vi "ZK非断电保存全局变量.vi"() -> ()   [LabVIEW 2022 SP3, in "质控单元V2.lvlib"]
uses:
  <vilib>/Plasmionique/MB Master/MB_Master/MB_Master.lvclass
panel:
  in  "静态加标设置":T1
  out "状态标记位_CODcr":bool
  out "状态标记位_CODMn":bool
  out "状态标记位_总氮":bool
  out "状态标记位_总磷":bool
  out "状态标记位_氨氮":bool
  in  "权限密码":u32[](array[numeric])=[0, 23506, 783523506, 783523103]
  in  "权限等级":enum16{"一级权限", "二级权限", "三级权限", "超级权限"}(ring)
  in  "CODCr运行模式":string
  in  "CODMn运行模式":string
  in  "总氮运行模式":string
  in  "总磷运行模式":string
  in  "氨氮运行模式":string
  in  "仪器状态显示":enum32{"氨氮", "总磷", "总氮", "CODmn", "CODcr"}(tab)
  in  "氨氮质控仪器状态显示":T2
  in  "总磷质控仪器状态显示":T2
  in  "总氮质控仪器状态显示":T2
  in  "CODMn质控仪器状态显示":T2
  in  "CODcr质控仪器状态显示":T2
  out "CODcr加标模块运行状态":string
  out "CODMn加标模块运行状态":string
  out "总氮加标模块运行状态":string
  out "总磷加标模块运行状态":string
  out "氨氮加标模块运行状态":string
  out "CODCr error out":errorcluster
  out "CODMn error out":errorcluster
  out "tn error out":errorcluster
  out "tp error out":errorcluster
  out "NH3N error out":errorcluster
  out "CODCr质控仪器状态":T3 {"当前步骤数" format="0x%04xH"}
  out "CODMn质控仪器状态":T3 {"当前步骤数" format="0x%04xH"}
  out "总氮质控仪器状态":T3 {"当前步骤数" format="0x%04xH"}
  out "总磷质控仪器状态":T3 {"当前步骤数" format="0x%04xH"}
  out "氨氮质控仪器状态":T3 {"当前步骤数" format="0x%04xH"}
  in  "ZK MB session in":refnum<class "MB_Master.lvclass">
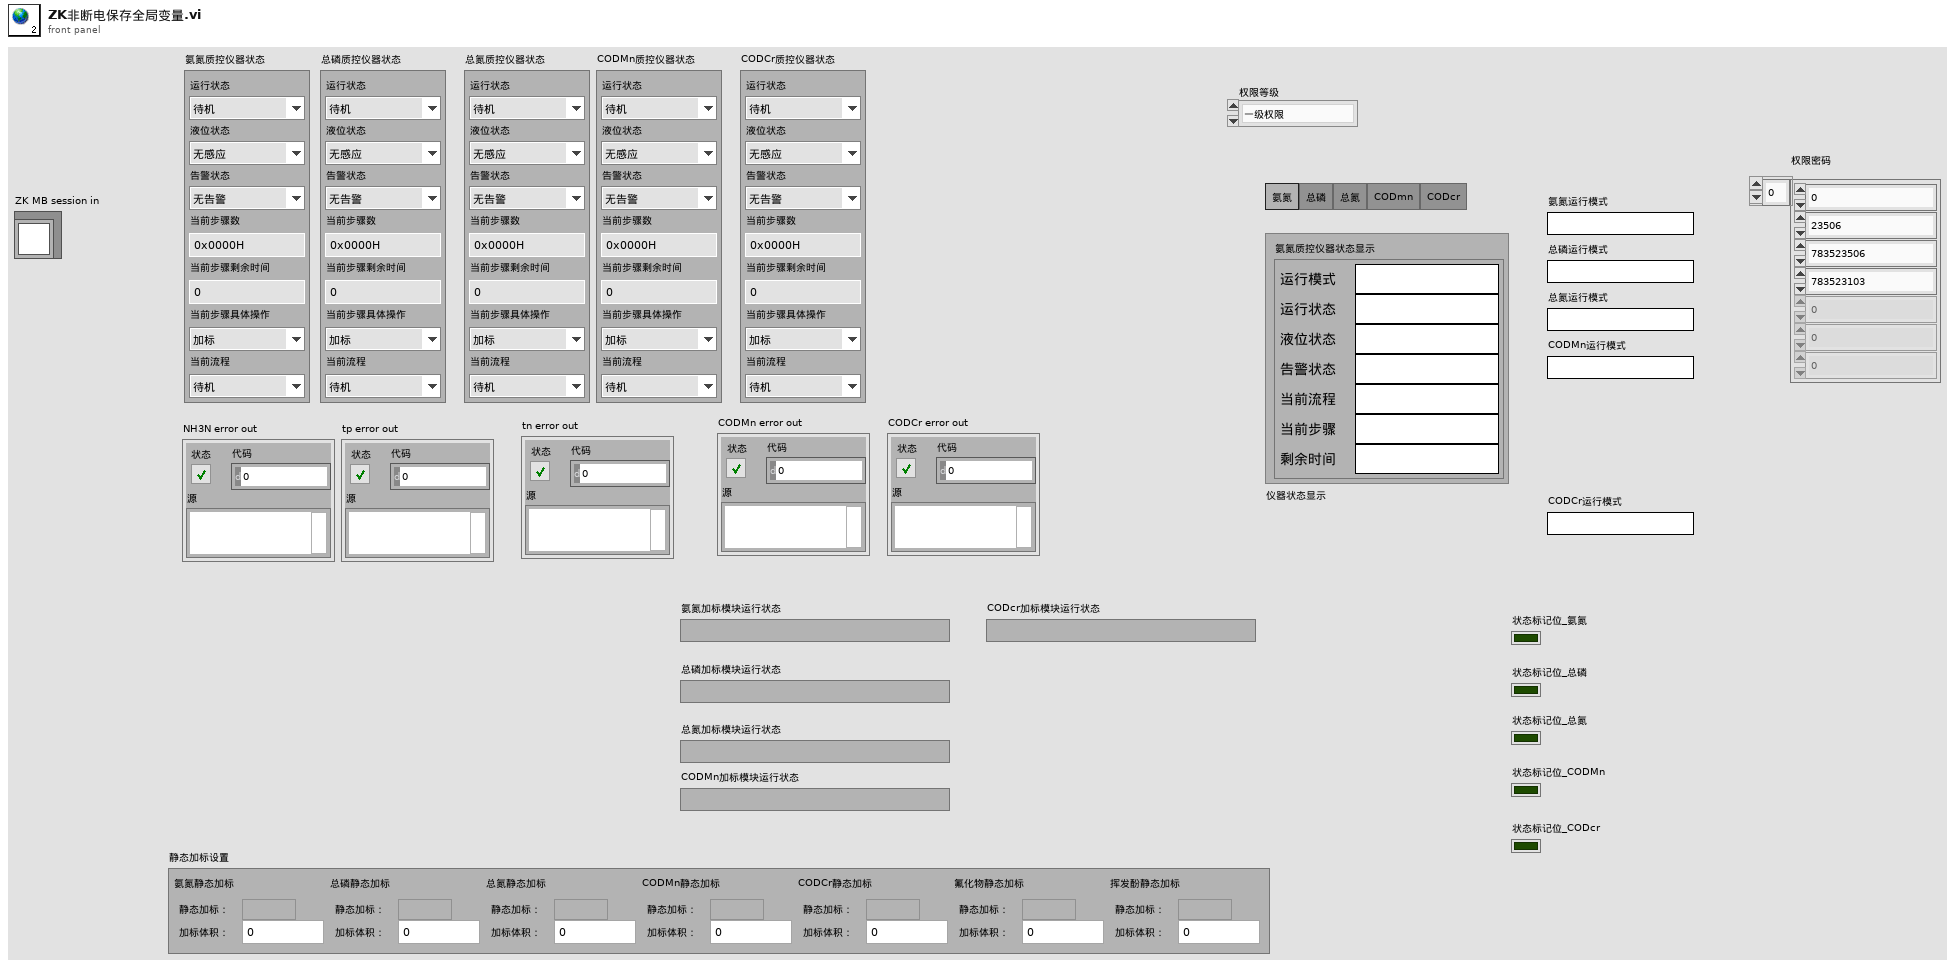
[diagram p1: front panel]
types:
  T1 = cluster{"氨氮静态加标":cluster{"静态加标：":bool, "加标体积":sgl}, "总磷静态加标":cluster{"静态加标：":bool, "加标体积":sgl}, "总氮静态加标":cluster{"静态加标：":bool, "加标体积":sgl}, "CODMn静态加标":cluster{"静态加标：":bool, "加标体积":sgl}, "CODCr静态加标":cluster{"静态加标：":bool, "加标体积":sgl}, "氟化物静态加标":cluster{"静态加标：":bool, "加标体积":sgl}, "挥发酚静态加标":cluster{"静态加标：":bool, "加标体积":sgl}}
  T2 = typedef "质控单元V2.lvlib/质控仪器状态显示.ctl" = cluster{"运行模式":string, "运行状态":string, "液位状态":string, "告警状态":string, "当前流程":string, "当前步骤":string, "剩余时间":string}
  T3 = typedef "质控单元V2.lvlib/质控仪器状态.ctl" = cluster{"运行状态":enum16{"待机", "润洗", "进样", "定量", "加标", "等待取样", "排液"}, "液位状态":enum16{"无感应", "有感应"}, "告警状态":enum16{"无告警", "液位故障告警", "注射泵异常"}, "当前步骤数":u16, "当前步骤剩余时间":u16, "当前步骤具体操作":enum16{"加标", "进样", "排液", "搅拌", "定量"}, "当前流程":enum16{"待机", "进样流程", "加标流程", "排液流程"}}
diagram:
